vi "DSF.Shared.Configuration.Transfer.Set Channel Blocks.vi"(10 "channel blocks":T1[](array[typedef]) {"buffer offset" format="%d bytes"}, 11 "Transfer Configuration in":refnum<class "DSF.Shared.Configuration.Transfer.lvclass">) -> (3 "Transfer Configuration out":refnum<class "DSF.Shared.Configuration.Transfer.lvclass">)   [LabVIEW 2017, in "DSF.Engine.lvlib" / "DSF.Shared.Configuration.Transfer.lvclass"]
uses:
  DSF.Shared.Configuration.Transfer.lvclass
  Typedefs/DSF.Shared.Refactor.Typedefs.Channel Block.ctl
  Typedefs/DSF.Shared.Typedefs.Data Type.ctl
  DSF.Shared.Configuration.Transfer.lvclass/DSF.Shared.Configuration.Transfer.ctl
  DSF.Engine.lvlib
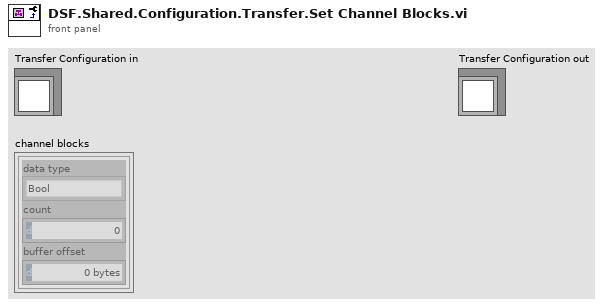
[diagram p1: front panel]
types:
  T1 = typedef "DSF.Engine.lvlib/DSF.Shared.Refactor.Typedefs.Channel Block.ctl" = cluster{"data type":T2, "count":u64, "buffer offset":u64}
  T2 = typedef "DSF.Shared.Typedefs.Data Type.ctl" = enum8{"Bool", "SGL", "DBL", "I8", "I16", "I32", "I64", "U8", "U16", "U32", "U64"}
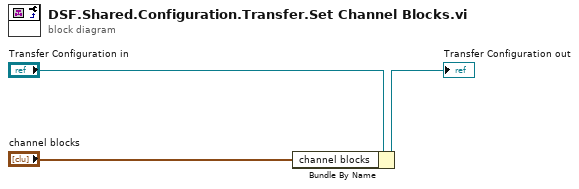
[diagram p0: block diagram]
diagram:
  n1 = Bundle By Name(cluster="Transfer Configuration in", "channel blocks"="channel blocks") -> (→"Transfer Configuration out":refnum<class "DSF.Shared.Configuration.Transfer.lvclass">)
